vi "Build.vi"(9 "XYZTheta":dbl[](array[numeric]), 10 "text file":dbl[][](array[numeric]), 11 "Sensor Dispense in":refnum<class "Sensor Dispense.lvclass">) -> (3 "Sensor Dispense out":refnum<class "Sensor Dispense.lvclass">)   [LabVIEW 2018, in "Sensor Dispense.lvclass"]
uses:
  Projects/Sensor Dispense.lvclass
  C:/Users/HEP/Documents/GitHub/New folder/C/Users/HEP/Documents/GitHub/UCSB-Gantry-HEP-2018/Classes/Routine/Dispense/Dispense.lvclass
  Projects/Sensor Dispense.lvclass/Sensor Dispense.ctl
  <vilib>/Analysis/coordinate.llb/2D Cartesian Coordinate Rotation (Scalar).vi
  <vilib>/Analysis/NI_AALPro.lvlib
panel:
  out "CW/CCW":dbl[](array[numeric])
  out "CW/CCW":dbl[](array[numeric])
  out "endpoints 2":dbl[][](array[numeric])
  out "endpoints":dbl[][](array[numeric])
  out "data":T1(array[cluster])
  out "cell count":dbl[](array[numeric])
  out "centers":dbl[][](array[numeric])
  # "[x1,y1,x2,y2]"
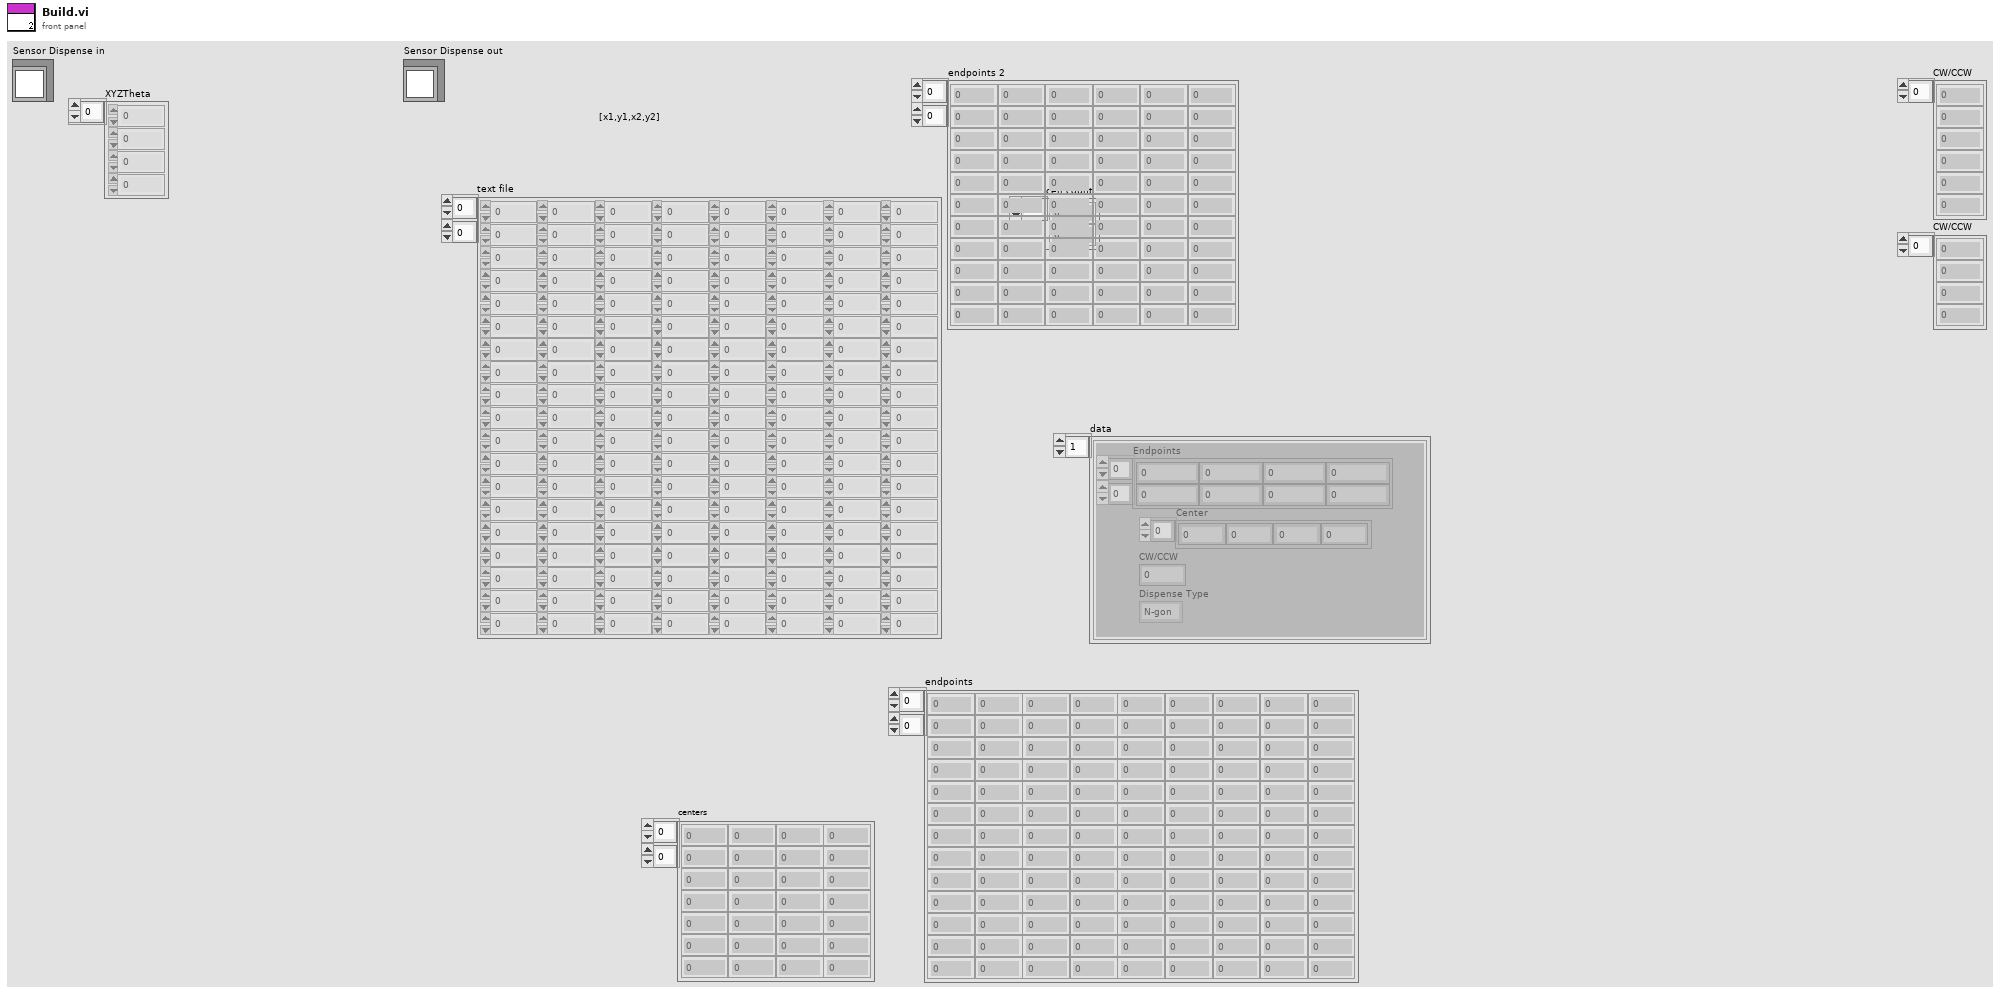
[diagram p1: front panel]
types:
  T1 = cluster{"Endpoints":dbl[][], "Center":dbl[], "CW/CCW":dbl, "Dispense Type":enum16{"N-gon", "Square", "Arc", "Dot", "Line", "Circle"}}[]
  T2 = enum16{"N-gon", "Square", "Arc", "Dot", "Line", "Circle"}
  T3 = cluster{"Endpoints":dbl[][], "Center":dbl[], "CW/CCW":dbl, "Dispense Type":enum16{"N-gon", "Square", "Arc", "Dot", "Line", "Circle"}}
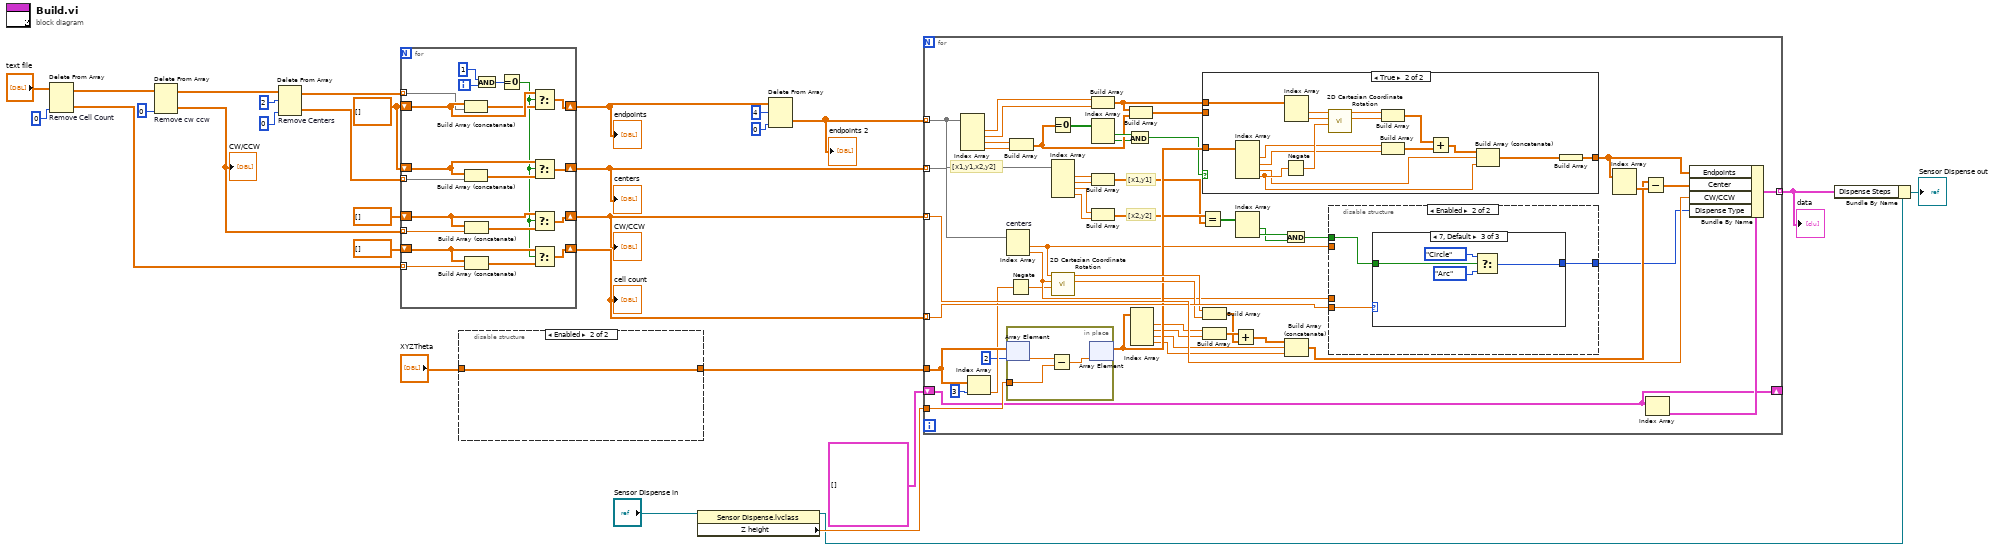
[diagram p0: block diagram]
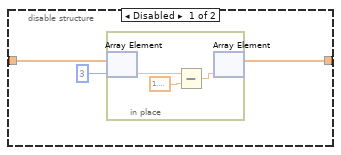
[diagram p2: hidden frame]
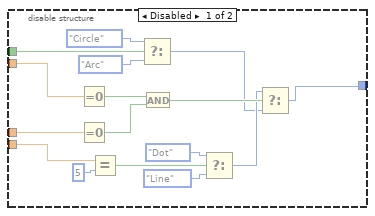
[diagram p3: hidden frame]
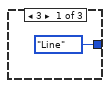
[diagram p4: hidden frame]
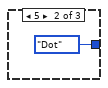
[diagram p5: hidden frame]
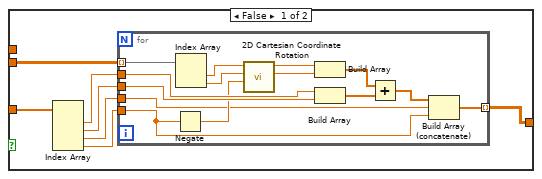
[diagram p6: hidden frame]
diagram:
  w26 = dbl[][] []
  n1 = Delete From Array "Remove Cell Count"(array="text file", index (col)=0) -> (deleted portion=w20:dbl[], array with subset deleted=w22:dbl[][])  [unwired: 2 in]
  n2 = Delete From Array "Remove cw ccw"(array=w22, index (col)=0 ("disabled index (col)")) -> (deleted portion=w2:dbl[], array with subset deleted=w19:dbl[][])  [unwired: 2 in]
  "CW/CCW" <- w2
  n3 = Delete From Array "Remove Centers"(array=w19, length=2, index (col)=0) -> (deleted portion=w15:dbl[][], array with subset deleted=w16:dbl[][])  [unwired: 1 in]
  n4 = for {
    tunnel: w16 -> [w45] mode=indexing
    shift-right: [w43] -> w9
    shift-left: w26 -> [w46]
    tunnel: w15 -> [w42] mode=indexing
    shift-right: [w39] -> w27
    shift-left: w26 -> [w40]
    tunnel: w20 -> [w38] mode=indexing
    shift-right: [w35] -> w24
    shift-left: dbl[] [] -> [w37]
    shift-right: [w30] -> w1
    shift-left: dbl[] [] -> [w33]
    tunnel: w2 -> [w34] mode=indexing
    i -> [w48]
    n5 = Build Array (concatenate)(w46, w45) -> (w44:dbl[][])
    n6 = Build Array (concatenate)(w40, w42) -> (w41:dbl[][])
    n7 = Build Array (concatenate)(w33, w34) -> (w32:dbl[])
    n8 = Build Array (concatenate)(w37, w38) -> (w36:dbl[])
    n9 = And(x=1, y=w48) -> (x .and. y?=w47:i32)
    n10 = Equal To 0?(x=w47) -> (x = 0?=w31:bool)
    n11 = Select(t=w46, s=w31, f=w44) -> (s? t:f=w43:dbl[][])
    n12 = Select(t=w40, s=w31, f=w41) -> (s? t:f=w39:dbl[][])
    n13 = Select(t=w33, s=w31, f=w32) -> (s? t:f=w30:dbl[])
    n14 = Select(t=w37, s=w31, f=w36) -> (s? t:f=w35:dbl[])
  }
  "centers" <- w27
  "cell count" <- w24
  "endpoints" <- w9
  "CW/CCW" <- w1
  n15 = disable-structure shown="Enabled" {
    disable-tunnel: "XYZTheta" -> [w52 w56]
    disable-tunnel: [w50 w56] -> w4
    frame Disabled {
      n16 = in-place {
        n17 = in-place-array #1(w52, 3) -> (w55:dbl)
        n18 = Subtract(x=w55, y=1.5707963267948966) -> (x-y=w53:dbl)
        n19 = in-place-array #1(w53) -> (w50:dbl[])  [unwired: 1 out]
      }
    }
    frame Enabled {
    }
  }
  n20 = property class="Sensor Dispense.lvclass"(reference="Sensor Dispense in") -> (reference out=w12:refnum<class "Sensor Dispense.lvclass">, "Z height"=w29:dbl)  [unwired: 1 in, 1 out]
  n21 = Delete From Array(array=w9, length=4, index (col)=0 ("disabled index (col)")) -> (deleted portion=w6:dbl[][])  [unwired: 1 in, 1 out]
  "endpoints 2" <- w6
  n22 = for {
    tunnel: w6 -> [w70] mode=indexing
    tunnel: w4 -> [w80]
    tunnel: w29 -> [w107]
    tunnel: w27 -> [w106] mode=indexing
    tunnel: w1 -> [w105] mode=indexing
    tunnel: w24 -> [w104] mode=indexing
    shift-right: [w89] -> _
    shift-left: T1 [] ("Dispense Steps") -> [w89]
    tunnel: [w103] -> w11 mode=indexing
    # "[x2,y2]"
    # "[x1,y1]"
    # "[x1,y1,x2,y2]"
    n23 = Index Array(array=w70) -> (element #1=w68:dbl, element #2=w67:dbl, element #3=w66:dbl, element #4=w65:dbl)  [unwired: 4 in]
    n24 = Index Array(array=w80, index=3) -> (element=w79:dbl)
    n25 = Index Array "centers"(array=w106) -> (element #1=w92:dbl, element #2=w91:dbl)  [unwired: 2 in]
    n26 = in-place {
      in-place-border: w107 -> [w134]
      n27 = in-place-array #2(w80, 2) -> (w135:dbl)
      n28 = Subtract(x=w135, y=w134) -> (x-y=w133:dbl)
      n29 = in-place-array #2(w133) -> (w100:dbl[])  [unwired: 1 out]
    }
    n30 = Negate(x=w79) -> (-x=w78:dbl)
    n31 = Build Array(w66, w65) -> (w62:dbl[])
    n32 = Equal To 0?(x=w62) -> (x = 0?=w61:bool[])
    n33 = Index Array(array=w70) -> (element #1=w76:dbl, element #2=w75:dbl, element #3=w88:dbl, element #4=w87:dbl)  [unwired: 4 in]
    n34 = call-poly <vilib>:"2D Cartesian Coordinate Rotation.vi"("theta"=w78, "y"=w91, "x"=w92) -> ("y out"=w101:dbl, "x out"=w102:dbl)  [unwired: 6 in, 1 out]
    n35 = Build Array(w68, w67) -> (w58:dbl[])
    n36 = Index Array(array=w61) -> (element #1=w63:bool, element #2=w59:bool)  [unwired: 2 in]
    n37 = Build Array(w76, w75) -> (w85:dbl[])
    n38 = Build Array(w88, w87) -> (w86:dbl[])
    n39 = And(x=w63, y=w59) -> (x .and. y?=w60:bool)
    n40 = Build Array(w58, w62) -> (w64:dbl[][])
    n41 = Index Array(array=w100) -> (element #1=w99:dbl, element #2=w96:dbl, element #3=w94:dbl, element #4=w93:dbl)  [unwired: 4 in]
    n42 = Equal?(x=w86, y=w85) -> (x = y?=w84:bool[])
    n43 = case shown="True" w60 {
      tunnel: w100 -> [w142 w169]
      tunnel: [w141 w157] -> w74
      tunnel: w64 -> [w140 _]
      tunnel: w58 -> [_ w172]
      frame False {
        n44 = Index Array(array=w142) -> (element #1=w139:dbl, element #2=w138:dbl, element #3=w136:dbl, element #4=w137:dbl)  [unwired: 4 in]
        n45 = for {
          tunnel: w140 -> [w156] mode=indexing
          tunnel: w139 -> [w153]
          tunnel: w138 -> [w152]
          tunnel: [w143] -> w141 mode=indexing
          tunnel: w137 -> [w144]
          tunnel: w136 -> [w145]
          n46 = Negate(x=w144) -> (-x=w147:dbl)
          n47 = Index Array(array=w156) -> (element #1=w155:dbl, element #2=w154:dbl)  [unwired: 2 in]
          n48 = call-poly <vilib>:"2D Cartesian Coordinate Rotation.vi"("theta"=w147, "y"=w154, "x"=w155) -> ("y out"=w150:dbl, "x out"=w151:dbl)  [unwired: 6 in, 1 out]
          n49 = Build Array(w151, w150) -> (w149:dbl[])
          n50 = Build Array(w153, w152) -> (w148:dbl[])
          n51 = Add(x=w149, y=w148) -> (x+y=w146:dbl[])
          n52 = Build Array (concatenate)(w146, w145, w144) -> (w143:dbl[])
        }
      }
      frame True {
        n53 = Index Array(array=w169) -> (element #1=w165:dbl, element #2=w164:dbl, element #3=w160:dbl, element #4=w161:dbl)  [unwired: 4 in]
        n54 = Negate(x=w161) -> (-x=w168:dbl)
        n55 = Index Array(array=w172) -> (element #1=w171:dbl, element #2=w170:dbl)  [unwired: 2 in]
        n56 = call-poly <vilib>:"2D Cartesian Coordinate Rotation.vi"("theta"=w168, "y"=w170, "x"=w171) -> ("y out"=w166:dbl, "x out"=w167:dbl)  [unwired: 6 in, 1 out]
        n57 = Build Array(w167, w166) -> (w162:dbl[])
        n58 = Build Array(w165, w164) -> (w163:dbl[])
        n59 = Add(x=w162, y=w163) -> (x+y=w159:dbl[])
        n60 = Build Array (concatenate)(w159, w160, w161) -> (w158:dbl[])
        n61 = Build Array(w158) -> (w157:dbl[][])
      }
    }
    n62 = Build Array(w102, w101) -> (w97:dbl[])
    n63 = Build Array(w99, w96) -> (w98:dbl[])
    n64 = Add(x=w98, y=w97) -> (x+y=w95:dbl[])
    n65 = Index Array(array=w84) -> (element #1=w82:bool, element #2=w83:bool)  [unwired: 2 in]
    n66 = And(x=w83, y=w82) -> (x .and. y?=w81:bool)
    n67 = Build Array (concatenate)(w95, w94, w93) -> (w72:dbl[])
    n68 = disable-structure shown="Enabled" {
      disable-tunnel: w104 -> [w123 w126]
      disable-tunnel: w92 -> [w120 _]
      disable-tunnel: w91 -> [w119 _]
      disable-tunnel: w81 -> [w112 w125]
      disable-tunnel: [w108 w124] -> w69
      frame Disabled {
        n69 = Equal To 0?(x=w120) -> (x = 0?=w121:bool)
        n70 = Equal To 0?(x=w119) -> (x = 0?=w122:bool)
        n71 = Equal?(x=w123, y=5) -> (x = y?=w115:bool)
        n72 = Select(t=T2."Circle" ("Dispense Type"), s=w112, f=T2."Arc" ("Dispense Type")) -> (s? t:f=w109:T2)
        n73 = And(x=w121, y=w122) -> (x .and. y?=w111:bool)
        n74 = Select(t=T2."Dot" ("Dispense Type"), s=w115, f=T2."Line" ("Dispense Type")) -> (s? t:f=w110:T2)
        n75 = Select(t=w110, s=w111, f=w109) -> (s? t:f=w108:T2)
      }
      frame Enabled {
        n76 = case shown="7, Default" w126 {
          tunnel: w125 -> [_ _ w130]
          tunnel: [T2."Line" ("Dispense Type") T2."Dot" ("Dispense Type") w129] -> w124
          frame 3 {
          }
          frame 5 {
          }
          frame 7, Default {
            n77 = Select(t=T2."Circle" ("Dispense Type"), s=w130, f=T2."Arc" ("Dispense Type")) -> (s? t:f=w129:T2)
          }
        }
      }
    }
    n78 = Index Array(array=w74) -> (element=w73:dbl[])  [unwired: 2 in]
    n79 = Subtract(x=w72, y=w73) -> (x-y=w71:dbl[])
    n80 = Index Array(array=w89) -> (element=w90:T3)  [unwired: 1 in]
    n81 = Bundle By Name(cluster=w90, "Endpoints"=w74, "Center"=w71, "CW/CCW"=w105, "Dispense Type"=w69) -> (w103:T3)
  }
  "data" <- w11
  n82 = Bundle By Name(cluster=w12, "Dispense Steps"=w11) -> (→"Sensor Dispense out":refnum<class "Sensor Dispense.lvclass">)
